vi "SAM.vi"() -> ()   [LabVIEW 2020]
uses:
  <vilib>/Utility/error.llb/DialogType.ctl
  <vilib>/DAQmx/read.llb/DAQmx Read (Analog 1D Wfm NChan NSamp).vi
  <vilib>/DAQmx/create/channels.llb/DAQmx Create Channel (AI-Voltage-Basic).vi
  <vilib>/DAQmx/configure/timing.llb/DAQmx Timing (Sample Clock).vi
  <vilib>/DAQmx/miscellaneous.llb/DAQmx Fill In Error Info.vi
  <vilib>/measure/matone.llb/Harmonic Distortion Analyzer 1 Chan.vi
  <vilib>/express/express analysis/Spectral/Block/exnSpectralBlock spectral measurements RMS poly.vi
  <vilib>/express/express analysis/Spectral/Block/exnSpectralBlock spectral measurements RMS WFM.vi
  <vilib>/measure/madcrms.llb/Basic Averaged DC-RMS for 1 Chan.vi
  <vilib>/measure/matone.llb/Extract Single Tone Information 1 Chan.vi
  <vilib>/express/express analysis/Spectral/XNode/ExpressSpectralMeasurementsBlockNode.xnode
  <resource>/objmgr/daqmx.rc
  <vilib>/measure/NI_MAPro.lvlib
panel:
  out "Voltage":waveform(dbl)(graph)
  out "Uc(Active Power)":dbl
  out "Active Power [W]":dbl
  out "Power":waveform(dbl)(graph)
  out "Phase dif.(V-I)":dbl
  out "THD(V) [dB]":dbl
  out "THD(I) [dB]":dbl
  out "Ih11 [dBA]":dbl
  out "Ih10 [dBA]":dbl
  out "Ih9 [dBA]":dbl
  out "Ih8 [dBA]":dbl
  out "Ih7 [dBA]":dbl
  out "Ih6 [dBA]":dbl
  out "Ih5 [dBA]":dbl
  out "Ih4 [dBA]":dbl
  out "Ih3 [dBA]":dbl
  out "Ih2 [dBA]":dbl
  out "Ih1 [dBA]":dbl
  out "Ih11 [A]":dbl
  out "Ih10 [A]":dbl
  out "Ih9 [A]":dbl
  out "Ih8 [A]":dbl
  out "Ih7 [A]":dbl
  out "Ih6 [A]":dbl
  out "Ih5 [A]":dbl
  out "Ih4 [A]":dbl
  out "Ih3 [A]":dbl
  out "Ih2 [A]":dbl
  out "Ih1 [A]":dbl
  out "fh(I)11 [Hz]":dbl
  out "fh(I)10 [Hz]":dbl
  out "fh(I)9 [Hz]":dbl
  out "fh(I)8 [Hz]":dbl
  out "fh(I)7 [Hz]":dbl
  out "fh(I)6 [Hz]":dbl
  out "fh(I)5 [Hz]":dbl
  out "fh(I)4 [Hz]":dbl
  out "fh(I)3 [Hz]":dbl
  out "fh(I)2 [Hz]":dbl
  out "fh(I)1 [Hz]":dbl
  out "Vh11 [dBV]":dbl
  out "Vh10 [dBV]":dbl
  out "Vh9 [dBV]":dbl
  out "Vh8 [dBV]":dbl
  out "Vh7 [dBV]":dbl
  out "Vh6 [dBV]":dbl
  out "Vh5 [dBV]":dbl
  out "Vh4 [dBV]":dbl
  out "Vh3 [dBV]":dbl
  out "Vh2 [dBV]":dbl
  out "Vh1 [dBV]":dbl
  out "Vh11 [V]":dbl
  out "Vh10 [V]":dbl
  out "Vh9 [V]":dbl
  out "Vh8 [V]":dbl
  out "Vh7 [V]":dbl
  out "Vh6 [V]":dbl
  out "Vh5 [V]":dbl
  out "Vh4 [V]":dbl
  out "Vh3 [V]":dbl
  out "Vh2 [V]":dbl
  out "Vh1 [V]":dbl
  out "fh(V)11 [Hz]":dbl
  out "fh(V)10 [Hz]":dbl
  out "fh(V)9 [Hz]":dbl
  out "fh(V)8 [Hz]":dbl
  out "fh(V)7 [Hz]":dbl
  out "fh(V)6 [Hz]":dbl
  out "fh(V)5 [Hz]":dbl
  out "fh(V)4 [Hz]":dbl
  out "fh(V)3 [Hz]":dbl
  out "fh(V)2 [Hz]":dbl
  out "fh(V)1 [Hz]":dbl
  out "One-sided Spectrum [dbV]":cluster{"f0":dbl, "df":dbl, "magnitude":dbl[]}(graph)
  out "One-sided Spectrum [dbA]":cluster{"f0":dbl, "df":dbl, "magnitude":dbl[]}(graph)
  out "Vrms(I) [A]":dbl
  out "Vm(I) [A]":dbl
  out "Vm(U) [V]":dbl
  out "Vrms(U) [V]":dbl
  out "f(I) [Hz]":dbl
  out "f(U) [Hz]":dbl
  out "Current":waveform(dbl)(graph)
  in  "stop":bool
  in  "Start":bool
  out "Actual sample clk  rate":dbl
  in  "sample clock source":tag
  in  "sample rate":dbl=1000.0 format="%0.2f"
  in  "n of samples":i32=1000
  in  "physical channel":tag
  in  "input terminal configuration":i32(ring)=-1 items=["Default"=-1, "RSE"=10083, "NRSE"=10078, "Differential"=10106, "Pseudodifferential"=12529]
  in  "Min V":dbl=-5.0 format="%0.2f"
  in  "Max V":dbl=5.0 format="%0.2f"
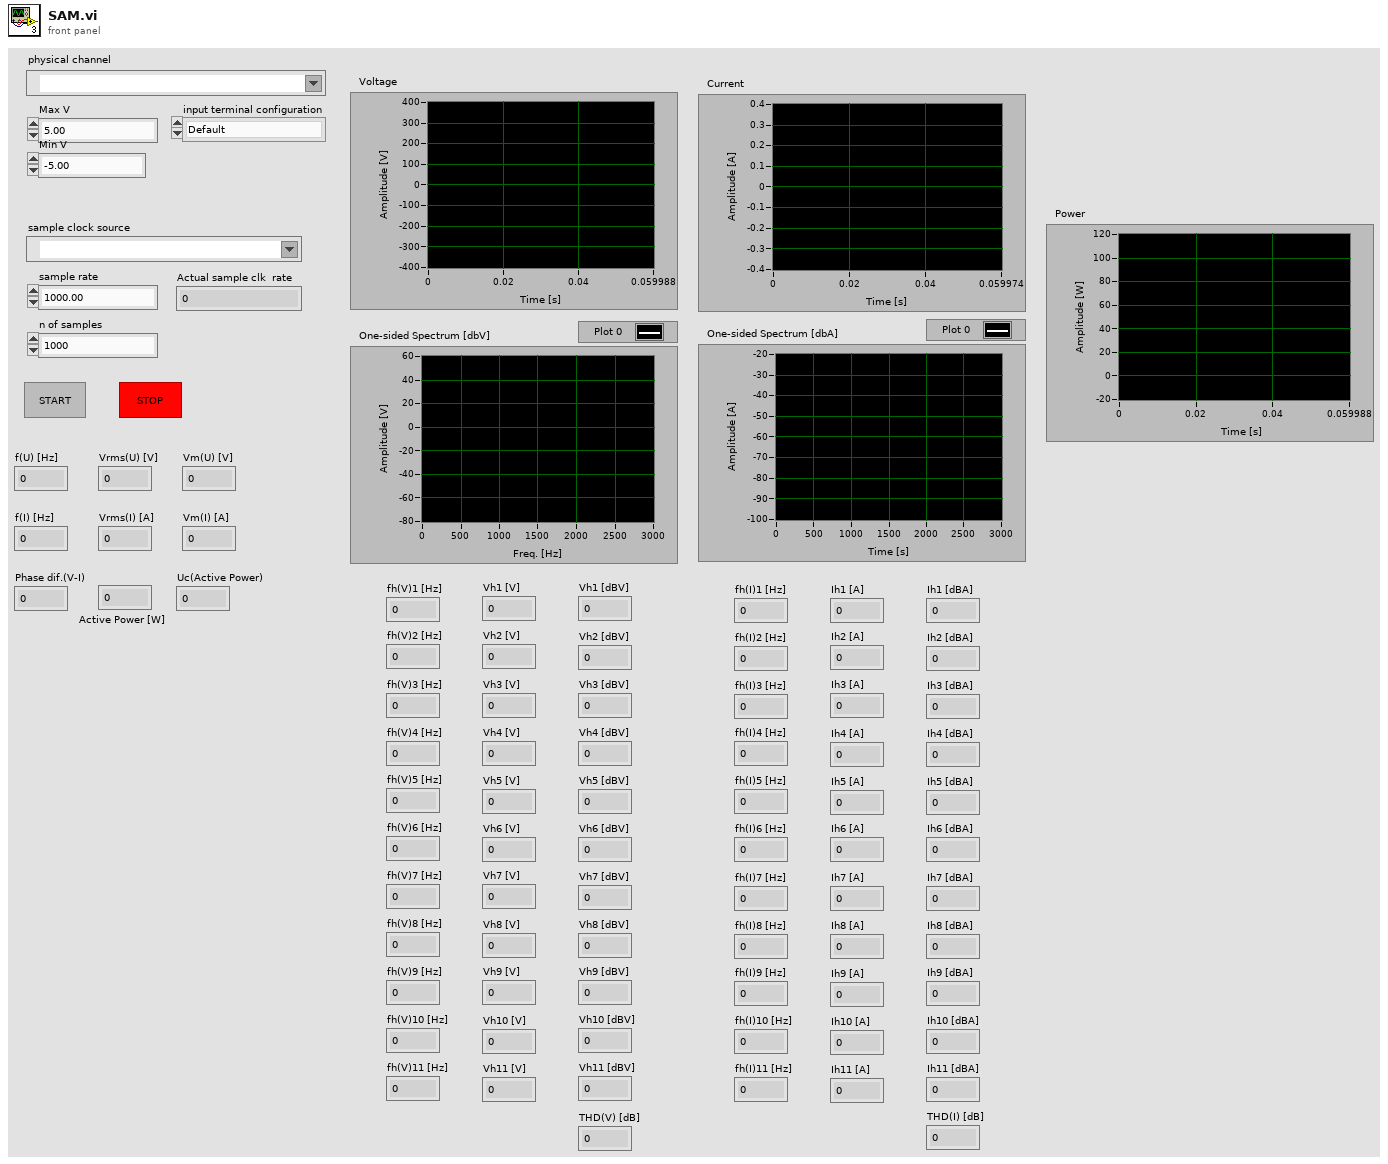
[diagram p1: front panel]
types:
  T1 = typedef "DialogType.ctl" = u16
  T2 = cluster{"averaging mode":u16, "weighting mode":u16, "number of averages":u32}
  T3 = cluster{"dB On (F)":bool, "unwrap phase (F)":bool, "convert to degree (F)":bool}
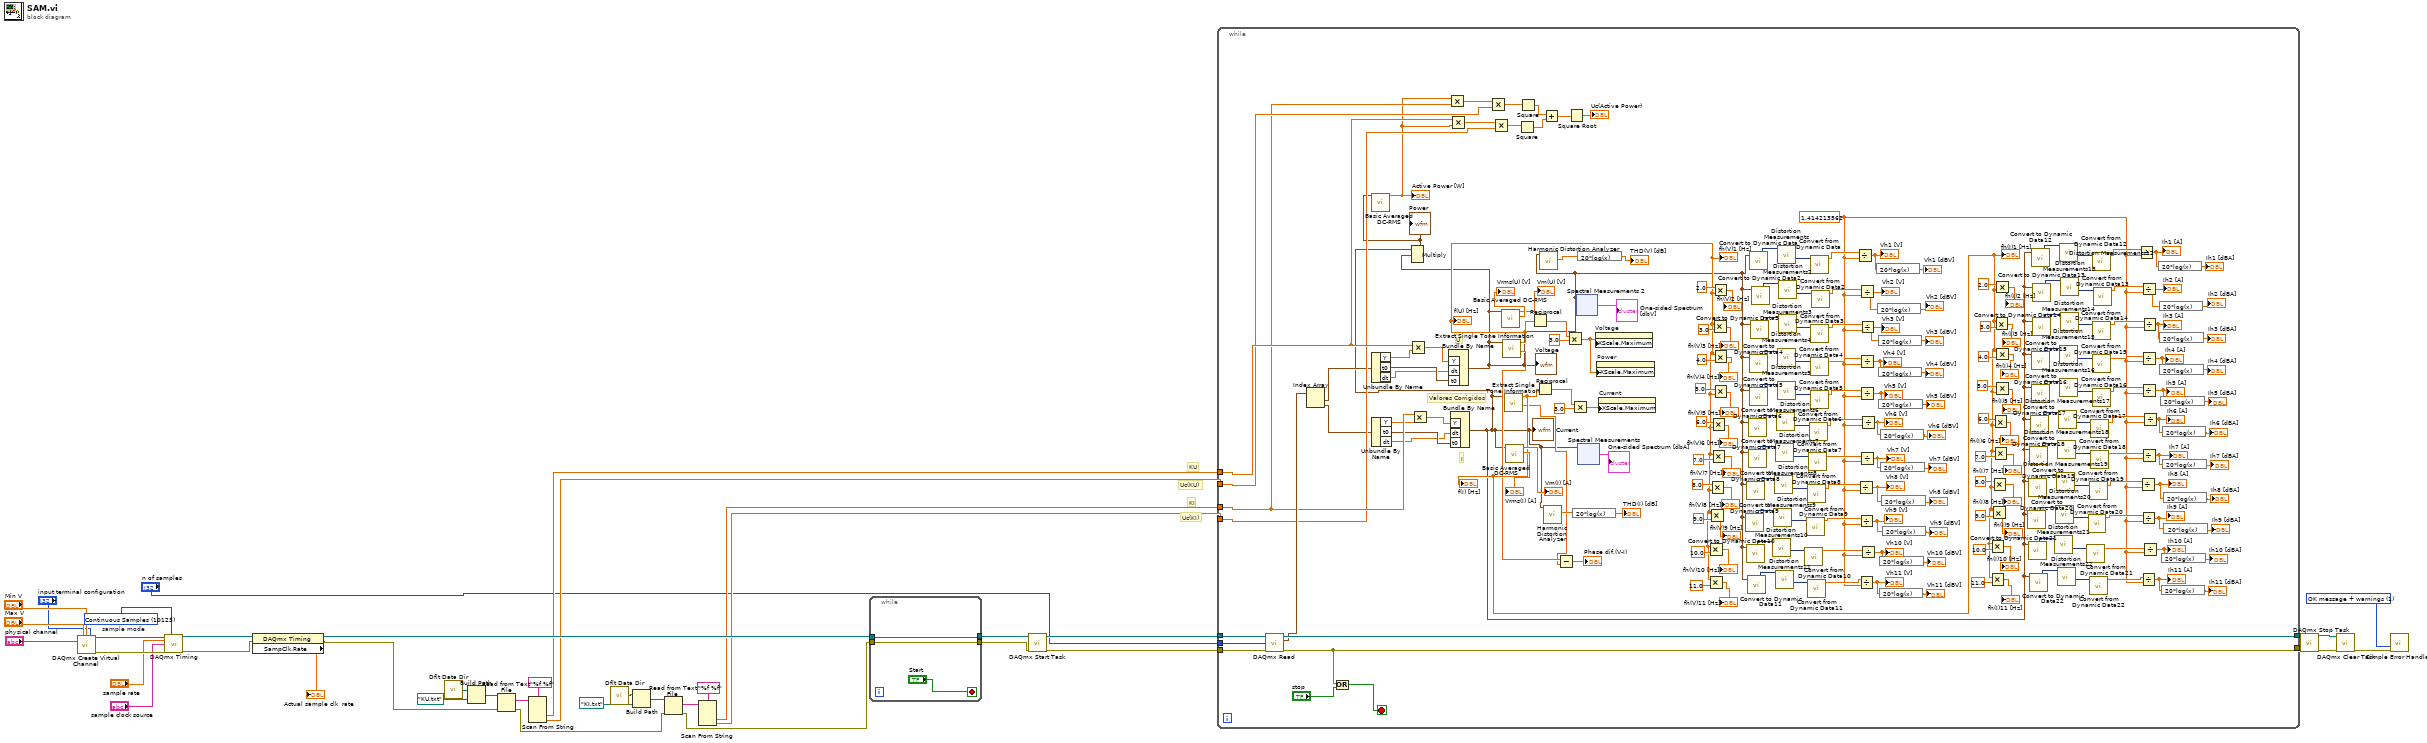
[diagram p0: block diagram]
diagram:
  w27 = T1 1 items=["no dialog", "OK message + warnings", "OK message", "continue or stop message", "continue/stop + warnings"] ("type of dialog (OK msg:1)")
  w33 = 10123 items=["Finite Samples"=10178, "Continuous Samples"=10123, "Hardware Timed Single Point"=12522]  # sample mode
  # "Uc(KU)"
  # "Uc(KI)"
  # "KI"
  # "KU"
  n1 = call-poly <vilib>:"DAQmx Create Virtual Channel.vi"("maximum value"="Max V", "minimum value"="Min V", "input terminal configuration"="input terminal configuration", "physical channels"="physical channel") -> ("task out"=w41:refnum<k21>, "error out"=w40:errorcluster)  [unwired: 10 in]
  n2 = call-poly <vilib>:"DAQmx Timing.vi"("task/channels in"=w41, "sample mode"=w33, "rate"="sample rate", "source"="sample clock source", "error in"=w40) -> ("task out"=w38:refnum<k21>, "error out"=w39:errorcluster)  [unwired: 9 in]
  n3 = property class="DAQmx Timing"(reference=w38, error in=w39) -> (reference out=w25:refnum<k21>, error out=w10:errorcluster, "SampClk.Rate"=→"Actual sample clk  rate":dbl)
  n4 = call <vilib>:"Dflt Data Dir.vi"() -> ("App:Default Data Directory"=w20:path)
  n5 = Build Path(base path=w20, name or relative path=path "KU.txt") -> (appended path=w16:path)
  n6 = Read from Text File(file (use dialog)=w16, error in=w10) -> (text=w17:string, error out=w9:errorcluster)  [unwired: 2 in, 2 out]
  n7 = Scan From String(format string="%f %f", input string=w17) -> (output 1=w7:dbl, output 2=w6:dbl)  [unwired: 4 in, 3 out]
  n8 = call <vilib>:"Dflt Data Dir.vi"() -> ("App:Default Data Directory"=w15:path)
  n9 = Build Path(base path=w15, name or relative path=path "KI.txt") -> (appended path=w11:path)
  n10 = Read from Text File(file (use dialog)=w11, error in=w9) -> (text=w12:string, error out=w8:errorcluster)  [unwired: 2 in, 2 out]
  n11 = Scan From String(format string="%f %f", input string=w12) -> (output 1=w5:dbl, output 2=w4:dbl)  [unwired: 4 in, 3 out]
  n12 = while {
    tunnel: w25 -> [w44]
    tunnel: [w44] -> w24
    tunnel: w8 -> [w43]
    tunnel: [w43] -> w23
    stop <- "Start" stop-if-true
  }
  n13 = call <vilib>:"DAQmx Start Task.vi"("task/channels in"=w24, "error in"=w23) -> ("task out"=w3:refnum<k21>, "error out"=w2:errorcluster)  [unwired: 12 in]
  n14 = while {
    tunnel: [w245] -> w22
    tunnel: [w246] -> w21
    tunnel: w7 -> [w243]
    tunnel: w6 -> [w242]
    tunnel: w5 -> [w241]
    tunnel: w4 -> [w240]
    tunnel: w3 -> [w248]
    tunnel: w2 -> [w247]
    tunnel: "n of samples" -> [w239]
    stop <- w249 stop-if-true
    w69 = 1.414213562 ("x")
    # "I"
    # "U"
    # "Valores Corrigidos"
    n15 = call-poly <vilib>:"DAQmx Read.vi"("task/channels in"=w248, "number of samples per channel"=w239, "error in"=w247) -> ("task out"=w246:refnum<k21>, "data"=w244:waveform(dbl)[], "error out"=w245:errorcluster)  [unwired: 10 in]
    n16 = Index Array(array=w244) -> (element #1=w238:waveform(dbl), element #2=w236:waveform(dbl))  [unwired: 2 in]
    n17 = Or(x=w245, y="stop") -> (x .or. y?=w249:bool)
    n18 = Unbundle By Name(w238) -> ("Y"=w232:dbl[], "t0"=w237:timestamp, "dt"=w233:dbl)
    n19 = Unbundle By Name(w236) -> ("Y"=w231:dbl[], "t0"=w235:timestamp, "dt"=w234:dbl)
    n20 = Multiply(x=w243, y=w232) -> (x*y=w229:dbl[])
    n21 = Multiply(x=w241, y=w231) -> (x*y=w230:dbl[])
    n22 = Bundle By Name("Y"=w229, "dt"=w233, "t0"=w237) -> (w46:waveform(dbl))  [unwired: 1 in]
    "Voltage" <- w46
    n23 = Bundle By Name("Y"=w230, "dt"=w234, "t0"=w235) -> (w59:waveform(dbl))  [unwired: 1 in]
    "Current" <- w59
    n24 = Multiply(1:w46, 2:w59) -> (0:w56:waveform(dbl))  [unwired: 1 in, 1 out]
    "Power" <- w56
    n25 = call-poly <vilib>:"Basic Averaged DC-RMS.vi"("signal in"=w56) -> ("DC value"=w47:dbl)  [unwired: 7 in, 3 out]
    "Active Power [W]" <- w47
    n26 = Multiply(x=w47, y=w241) -> (x*y=w49:dbl)
    n27 = Multiply(x=w243, y=w47) -> (x*y=w48:dbl)
    n28 = Multiply(x=w49, y=w242) -> (x*y=w51:dbl)
    n29 = Multiply(x=w48, y=w240) -> (x*y=w50:dbl)
    n30 = call-poly <vilib>:"Basic Averaged DC-RMS.vi"("signal in"=w46) -> ("RMS value"=→"Vrms(U) [V]":dbl, "DC value"=→"Vm(U) [V]":dbl)  [unwired: 7 in, 2 out]
    n31 = call-poly <vilib>:"Extract Single Tone Information.vi"("time signal in"=w46) -> ("detected phase (deg)"=w62:dbl, "detected frequency"=w185:dbl)  [unwired: 5 in, 4 out]
    "f(U) [Hz]" <- w185
    "fh(V)1 [Hz]" <- w185
    n32 = call-poly <vilib>:"Extract Single Tone Information.vi"("time signal in"=w59) -> ("detected phase (deg)"=w61:dbl, "detected frequency"=w68:dbl)  [unwired: 5 in, 4 out]
    "f(I) [Hz]" <- w68
    "fh(I)1 [Hz]" <- w68
    n33 = call-poly <vilib>:"Basic Averaged DC-RMS.vi"("signal in"=w59) -> ("RMS value"=→"Vrms(I) [A]":dbl, "DC value"=→"Vm(I) [A]":dbl)  [unwired: 7 in, 2 out]
    n34 = Square(x=w50) -> (x^2=w52:dbl)
    n35 = Square(x=w51) -> (x^2=w53:dbl)
    n36 = Reciprocal(x=w185) -> (1/x=w228:dbl)
    n37 = Reciprocal(x=w68) -> (1/x=w226:dbl)
    n38 = call-poly <vilib>:"Harmonic Distortion Analyzer.vi"("signal in"=w46) -> ("THD"=w67:dbl)  [unwired: 5 in, 5 out]
    n39 = Add(x=w53, y=w52) -> (x+y=w54:dbl)
    n40 = call-poly <vilib>:"Harmonic Distortion Analyzer.vi"("signal in"=w59) -> ("THD"=w66:dbl)  [unwired: 5 in, 5 out]
    n41 = Subtract(x=w62, y=w61) -> (x-y=→"Phase dif.(V-I)":dbl)
    n42 = Multiply(x=w228, y=3.0 ("x*y")) -> (x*y=w45:dbl)
    n43 = Square Root(x=w54) -> (sqrt(x)=→"Uc(Active Power)":dbl)
    n44 = Multiply(x=w226, y=3.0 ("x*y")) -> (x*y=w224:dbl)
    n45 = expression code="20*log(x)"(w66) -> (→"THD(I) [dB]":dbl)
    n46 = xnode "Spectral Measurements 2"("Signals"=w46) -> ("FFT - (RMS)"=→"One-sided Spectrum [dbV]":cluster{"f0":dbl, "df":dbl, "magnitude":dbl[]})  [unwired: 1 in, 2 out]
    n47 = expression code="20*log(x)"(w67) -> (→"THD(V) [dB]":dbl)
    n48 = xnode "Spectral Measurements"("Signals"=w59) -> ("FFT - (RMS)"=→"One-sided Spectrum [dbA]":cluster{"f0":dbl, "df":dbl, "magnitude":dbl[]})  [unwired: 1 in, 2 out]
    n49 = property on="Voltage" class="WFGraph (strict)"("XScale.Maximum"=w45) -> ()  [unwired: 2 in, 2 out]
    n50 = property on="Power" class="WFGraph (strict)"("XScale.Maximum"=w45) -> ()  [unwired: 2 in, 2 out]
    n51 = property on="Current" class="WFGraph (strict)"("XScale.Maximum"=w224) -> ()  [unwired: 2 in, 2 out]
    n52 = Multiply(x=w185, y=10.0) -> (x*y=→"fh(V)10 [Hz]":dbl)
    n53 = Multiply(x=w185, y=11.0) -> (x*y=→"fh(V)11 [Hz]":dbl)
    n54 = Multiply(x=w185, y=9.0 ("x*y")) -> (x*y=→"fh(V)9 [Hz]":dbl)
    n55 = Multiply(x=8.0, y=w185) -> (x*y=→"fh(V)8 [Hz]":dbl)
    n56 = Multiply(x=6.0 ("x*y"), y=w185) -> (x*y=→"fh(V)6 [Hz]":dbl)
    n57 = Multiply(x=w185, y=7.0) -> (x*y=→"fh(V)7 [Hz]":dbl)
    n58 = Multiply(x=w185, y=3.0 ("x*y")) -> (x*y=→"fh(V)3 [Hz]":dbl)
    n59 = Multiply(x=2.0, y=w185) -> (x*y=→"fh(V)2 [Hz]":dbl)
    n60 = Multiply(x=w185, y=4.0 ("x*y")) -> (x*y=→"fh(V)4 [Hz]":dbl)
    n61 = Multiply(x=5.0, y=w185) -> (x*y=→"fh(V)5 [Hz]":dbl)
    n62 = call "Convert to Dynamic Data9"("Waveform"=w46) -> ("Dynamic Data Type"=w201:dynamicdata)  [unwired: 3 in]
    n63 = call "Convert to Dynamic Data10"("Waveform"=w46) -> ("Dynamic Data Type"=w198:dynamicdata)  [unwired: 3 in]
    n64 = call "Convert to Dynamic Data8"("Waveform"=w46) -> ("Dynamic Data Type"=w202:dynamicdata)  [unwired: 3 in]
    n65 = call "Convert to Dynamic Data11"("Waveform"=w46) -> ("Dynamic Data Type"=w197:dynamicdata)  [unwired: 3 in]
    n66 = call "Convert to Dynamic Data7"("Waveform"=w46) -> ("Dynamic Data Type"=w205:dynamicdata)  [unwired: 3 in]
    n67 = call "Convert to Dynamic Data6"("Waveform"=w46) -> ("Dynamic Data Type"=w206:dynamicdata)  [unwired: 3 in]
    n68 = call "Convert to Dynamic Data"("Waveform"=w46) -> ("Dynamic Data Type"=w217:dynamicdata)  [unwired: 3 in]
    n69 = call "Convert to Dynamic Data4"("Waveform"=w46) -> ("Dynamic Data Type"=w210:dynamicdata)  [unwired: 3 in]
    n70 = call "Convert to Dynamic Data5"("Waveform"=w46) -> ("Dynamic Data Type"=w209:dynamicdata)  [unwired: 3 in]
    n71 = call "Convert to Dynamic Data3"("Waveform"=w46) -> ("Dynamic Data Type"=w213:dynamicdata)  [unwired: 3 in]
    n72 = call "Convert to Dynamic Data2"("Waveform"=w46) -> ("Dynamic Data Type"=w214:dynamicdata)  [unwired: 3 in]
    n73 = call "Distortion Measurements10"("Signals"=w198) -> ("Specific Harmonic"=w199:dynamicdata)  [unwired: 9 in, 1 out]
    n74 = call "Distortion Measurements9"("Signals"=w201) -> ("Specific Harmonic"=w200:dynamicdata)  [unwired: 9 in, 1 out]
    n75 = call "Distortion Measurements8"("Signals"=w202) -> ("Specific Harmonic"=w203:dynamicdata)  [unwired: 9 in, 1 out]
    n76 = call "Distortion Measurements11"("Signals"=w197) -> ("Specific Harmonic"=w196:dynamicdata)  [unwired: 9 in, 1 out]
    n77 = call "Distortion Measurements7"("Signals"=w205) -> ("Specific Harmonic"=w204:dynamicdata)  [unwired: 9 in, 1 out]
    n78 = call "Distortion Measurements6"("Signals"=w206) -> ("Specific Harmonic"=w207:dynamicdata)  [unwired: 9 in, 1 out]
    n79 = call "Distortion Measurements"("Signals"=w217) -> ("Specific Harmonic"=w216:dynamicdata)  [unwired: 9 in, 1 out]
    n80 = call "Distortion Measurements4"("Signals"=w210) -> ("Specific Harmonic"=w211:dynamicdata)  [unwired: 9 in, 1 out]
    n81 = call "Distortion Measurements5"("Signals"=w209) -> ("Specific Harmonic"=w208:dynamicdata)  [unwired: 9 in, 1 out]
    n82 = call "Distortion Measurements3"("Signals"=w213) -> ("Specific Harmonic"=w212:dynamicdata)  [unwired: 9 in, 1 out]
    n83 = call "Distortion Measurements2"("Signals"=w214) -> ("Specific Harmonic"=w215:dynamicdata)  [unwired: 9 in, 1 out]
    n84 = call "Convert from Dynamic Data10"("Dynamic Data Type"=w199) -> ("Scalar"=w165:dbl)  [unwired: 3 in]
    n85 = call "Convert from Dynamic Data9"("Dynamic Data Type"=w200) -> ("Scalar"=w166:dbl)  [unwired: 3 in]
    n86 = call "Convert from Dynamic Data8"("Dynamic Data Type"=w203) -> ("Scalar"=w167:dbl)  [unwired: 3 in]
    n87 = call "Convert from Dynamic Data11"("Dynamic Data Type"=w196) -> ("Scalar"=w164:dbl)  [unwired: 3 in]
    n88 = call "Convert from Dynamic Data7"("Dynamic Data Type"=w204) -> ("Scalar"=w168:dbl)  [unwired: 3 in]
    n89 = call "Convert from Dynamic Data6"("Dynamic Data Type"=w207) -> ("Scalar"=w169:dbl)  [unwired: 3 in]
    n90 = call "Convert from Dynamic Data"("Dynamic Data Type"=w216) -> ("Scalar"=w174:dbl)  [unwired: 3 in]
    n91 = call "Convert from Dynamic Data4"("Dynamic Data Type"=w211) -> ("Scalar"=w171:dbl)  [unwired: 3 in]
    n92 = call "Convert from Dynamic Data5"("Dynamic Data Type"=w208) -> ("Scalar"=w170:dbl)  [unwired: 3 in]
    n93 = call "Convert from Dynamic Data3"("Dynamic Data Type"=w212) -> ("Scalar"=w172:dbl)  [unwired: 3 in]
    n94 = call "Convert from Dynamic Data2"("Dynamic Data Type"=w215) -> ("Scalar"=w173:dbl)  [unwired: 3 in]
    n95 = Divide(x=w174, y=w69) -> (x/y=w163:dbl)
    "Vh1 [V]" <- w163
    n96 = Divide(x=w167, y=w69) -> (x/y=w57:dbl)
    "Vh8 [V]" <- w57
    n97 = Divide(x=w166, y=w69) -> (x/y=w152:dbl)
    "Vh9 [V]" <- w152
    n98 = Divide(x=w164, y=w69) -> (x/y=w150:dbl)
    "Vh11 [V]" <- w150
    n99 = Divide(x=w173, y=w69) -> (x/y=w160:dbl)
    "Vh2 [V]" <- w160
    n100 = Divide(x=w171, y=w69) -> (x/y=w156:dbl)
    "Vh4 [V]" <- w156
    n101 = Divide(x=w170, y=w69) -> (x/y=w154:dbl)
    "Vh5 [V]" <- w154
    n102 = Divide(x=w168, y=w69) -> (x/y=w153:dbl)
    "Vh7 [V]" <- w153
    n103 = Divide(x=w172, y=w69) -> (x/y=w158:dbl)
    "Vh3 [V]" <- w158
    n104 = Divide(x=w169, y=w69) -> (x/y=w149:dbl)
    "Vh6 [V]" <- w149
    n105 = Divide(x=w165, y=w69) -> (x/y=w151:dbl)
    "Vh10 [V]" <- w151
    n106 = expression code="20*log(x)"(w163) -> (→"Vh1 [dBV]":dbl)
    n107 = expression code="20*log(x)"(w160) -> (→"Vh2 [dBV]":dbl)
    n108 = expression code="20*log(x)"(w158) -> (→"Vh3 [dBV]":dbl)
    n109 = expression code="20*log(x)"(w156) -> (→"Vh4 [dBV]":dbl)
    n110 = expression code="20*log(x)"(w154) -> (→"Vh5 [dBV]":dbl)
    n111 = expression code="20*log(x)"(w150) -> (→"Vh11 [dBV]":dbl)
    n112 = expression code="20*log(x)"(w151) -> (→"Vh10 [dBV]":dbl)
    n113 = expression code="20*log(x)"(w149) -> (→"Vh6 [dBV]":dbl)
    n114 = expression code="20*log(x)"(w153) -> (→"Vh7 [dBV]":dbl)
    n115 = expression code="20*log(x)"(w57) -> (→"Vh8 [dBV]":dbl)
    n116 = expression code="20*log(x)"(w152) -> (→"Vh9 [dBV]":dbl)
    n117 = Multiply(x=w68, y=10.0) -> (x*y=→"fh(I)10 [Hz]":dbl)
    n118 = Multiply(x=w68, y=11.0) -> (x*y=→"fh(I)11 [Hz]":dbl)
    n119 = Multiply(x=w68, y=9.0 ("x*y")) -> (x*y=→"fh(I)9 [Hz]":dbl)
    n120 = Multiply(x=8.0 ("y"), y=w68) -> (x*y=→"fh(I)8 [Hz]":dbl)
    n121 = Multiply(x=6.0 ("x*y"), y=w68) -> (x*y=→"fh(I)6 [Hz]":dbl)
    n122 = Multiply(x=w68, y=7.0) -> (x*y=→"fh(I)7 [Hz]":dbl)
    n123 = Multiply(x=w68, y=3.0 ("x*y")) -> (x*y=→"fh(I)3 [Hz]":dbl)
    n124 = Multiply(x=2.0, y=w68) -> (x*y=→"fh(I)2 [Hz]":dbl)
    n125 = Multiply(x=w68, y=4.0 ("x*y")) -> (x*y=→"fh(I)4 [Hz]":dbl)
    n126 = Multiply(x=5.0, y=w68) -> (x*y=→"fh(I)5 [Hz]":dbl)
    n127 = call "Convert to Dynamic Data20"("Waveform"=w59) -> ("Dynamic Data Type"=w126:dynamicdata)  [unwired: 3 in]
    n128 = call "Convert to Dynamic Data21"("Waveform"=w59) -> ("Dynamic Data Type"=w123:dynamicdata)  [unwired: 3 in]
    n129 = call "Convert to Dynamic Data19"("Waveform"=w59) -> ("Dynamic Data Type"=w127:dynamicdata)  [unwired: 3 in]
    n130 = call "Convert to Dynamic Data22"("Waveform"=w59) -> ("Dynamic Data Type"=w122:dynamicdata)  [unwired: 3 in]
    n131 = call "Convert to Dynamic Data18"("Waveform"=w59) -> ("Dynamic Data Type"=w130:dynamicdata)  [unwired: 3 in]
    n132 = call "Convert to Dynamic Data17"("Waveform"=w59) -> ("Dynamic Data Type"=w131:dynamicdata)  [unwired: 3 in]
    n133 = call "Convert to Dynamic Data12"("Waveform"=w59) -> ("Dynamic Data Type"=w142:dynamicdata)  [unwired: 3 in]
    n134 = call "Convert to Dynamic Data15"("Waveform"=w59) -> ("Dynamic Data Type"=w135:dynamicdata)  [unwired: 3 in]
    n135 = call "Convert to Dynamic Data16"("Waveform"=w59) -> ("Dynamic Data Type"=w134:dynamicdata)  [unwired: 3 in]
    n136 = call "Convert to Dynamic Data14"("Waveform"=w59) -> ("Dynamic Data Type"=w138:dynamicdata)  [unwired: 3 in]
    n137 = call "Convert to Dynamic Data13"("Waveform"=w59) -> ("Dynamic Data Type"=w139:dynamicdata)  [unwired: 3 in]
    n138 = call "Distortion Measurements21"("Signals"=w123) -> ("Specific Harmonic"=w124:dynamicdata)  [unwired: 9 in, 1 out]
    n139 = call "Distortion Measurements20"("Signals"=w126) -> ("Specific Harmonic"=w125:dynamicdata)  [unwired: 9 in, 1 out]
    n140 = call "Distortion Measurements19"("Signals"=w127) -> ("Specific Harmonic"=w128:dynamicdata)  [unwired: 9 in, 1 out]
    n141 = call "Distortion Measurements22"("Signals"=w122) -> ("Specific Harmonic"=w121:dynamicdata)  [unwired: 9 in, 1 out]
    n142 = call "Distortion Measurements18"("Signals"=w130) -> ("Specific Harmonic"=w129:dynamicdata)  [unwired: 9 in, 1 out]
    n143 = call "Distortion Measurements17"("Signals"=w131) -> ("Specific Harmonic"=w132:dynamicdata)  [unwired: 9 in, 1 out]
    n144 = call "Distortion Measurements12"("Signals"=w142) -> ("Specific Harmonic"=w141:dynamicdata)  [unwired: 9 in, 1 out]
    n145 = call "Distortion Measurements15"("Signals"=w135) -> ("Specific Harmonic"=w136:dynamicdata)  [unwired: 9 in, 1 out]
    n146 = call "Distortion Measurements16"("Signals"=w134) -> ("Specific Harmonic"=w133:dynamicdata)  [unwired: 9 in, 1 out]
    n147 = call "Distortion Measurements14"("Signals"=w138) -> ("Specific Harmonic"=w137:dynamicdata)  [unwired: 9 in, 1 out]
    n148 = call "Distortion Measurements13"("Signals"=w139) -> ("Specific Harmonic"=w140:dynamicdata)  [unwired: 9 in, 1 out]
    n149 = call "Convert from Dynamic Data21"("Dynamic Data Type"=w124) -> ("Scalar"=w92:dbl)  [unwired: 3 in]
    n150 = call "Convert from Dynamic Data20"("Dynamic Data Type"=w125) -> ("Scalar"=w93:dbl)  [unwired: 3 in]
    n151 = call "Convert from Dynamic Data19"("Dynamic Data Type"=w128) -> ("Scalar"=w94:dbl)  [unwired: 3 in]
    n152 = call "Convert from Dynamic Data22"("Dynamic Data Type"=w121) -> ("Scalar"=w91:dbl)  [unwired: 3 in]
    n153 = call "Convert from Dynamic Data18"("Dynamic Data Type"=w129) -> ("Scalar"=w95:dbl)  [unwired: 3 in]
    n154 = call "Convert from Dynamic Data17"("Dynamic Data Type"=w132) -> ("Scalar"=w96:dbl)  [unwired: 3 in]
    n155 = call "Convert from Dynamic Data12"("Dynamic Data Type"=w141) -> ("Scalar"=w101:dbl)  [unwired: 3 in]
    n156 = call "Convert from Dynamic Data15"("Dynamic Data Type"=w136) -> ("Scalar"=w98:dbl)  [unwired: 3 in]
    n157 = call "Convert from Dynamic Data16"("Dynamic Data Type"=w133) -> ("Scalar"=w97:dbl)  [unwired: 3 in]
    n158 = call "Convert from Dynamic Data14"("Dynamic Data Type"=w137) -> ("Scalar"=w99:dbl)  [unwired: 3 in]
    n159 = call "Convert from Dynamic Data13"("Dynamic Data Type"=w140) -> ("Scalar"=w100:dbl)  [unwired: 3 in]
    n160 = Divide(x=w101, y=w69) -> (x/y=w90:dbl)
    "Ih1 [A]" <- w90
    n161 = Divide(x=w94, y=w69) -> (x/y=w58:dbl)
    "Ih8 [A]" <- w58
    n162 = Divide(x=w93, y=w69) -> (x/y=w79:dbl)
    "Ih9 [A]" <- w79
    n163 = Divide(x=w91, y=w69) -> (x/y=w77:dbl)
    "Ih11 [A]" <- w77
    n164 = Divide(x=w100, y=w69) -> (x/y=w87:dbl)
    "Ih2 [A]" <- w87
    n165 = Divide(x=w98, y=w69) -> (x/y=w83:dbl)
    "Ih4 [A]" <- w83
    n166 = Divide(x=w97, y=w69) -> (x/y=w81:dbl)
    "Ih5 [A]" <- w81
    n167 = Divide(x=w95, y=w69) -> (x/y=w80:dbl)
    "Ih7 [A]" <- w80
    n168 = Divide(x=w99, y=w69) -> (x/y=w85:dbl)
    "Ih3 [A]" <- w85
    n169 = Divide(x=w96, y=w69) -> (x/y=w76:dbl)
    "Ih6 [A]" <- w76
    n170 = Divide(x=w92, y=w69) -> (x/y=w78:dbl)
    "Ih10 [A]" <- w78
    n171 = expression code="20*log(x)"(w90) -> (→"Ih1 [dBA]":dbl)
    n172 = expression code="20*log(x)"(w87) -> (→"Ih2 [dBA]":dbl)
    n173 = expression code="20*log(x)"(w85) -> (→"Ih3 [dBA]":dbl)
    n174 = expression code="20*log(x)"(w83) -> (→"Ih4 [dBA]":dbl)
    n175 = expression code="20*log(x)"(w81) -> (→"Ih5 [dBA]":dbl)
    n176 = expression code="20*log(x)"(w77) -> (→"Ih11 [dBA]":dbl)
    n177 = expression code="20*log(x)"(w78) -> (→"Ih10 [dBA]":dbl)
    n178 = expression code="20*log(x)"(w76) -> (→"Ih6 [dBA]":dbl)
    n179 = expression code="20*log(x)"(w80) -> (→"Ih7 [dBA]":dbl)
    n180 = expression code="20*log(x)"(w58) -> (→"Ih8 [dBA]":dbl)
    n181 = expression code="20*log(x)"(w79) -> (→"Ih9 [dBA]":dbl)
  }
  n182 = call <vilib>:"DAQmx Stop Task.vi"("task/channels in"=w21, "error in"=w22) -> ("task out"=w30:refnum<k21>, "error out"=w29:errorcluster)  [unwired: 12 in]
  n183 = call <vilib>:"DAQmx Clear Task.vi"("task in"=w30, "error in"=w29) -> ("error out"=w28:errorcluster)  [unwired: 13 in]
  n184 = call <vilib>:"Simple Error Handler.vi"("type of dialog (OK msg:1)"=w27, "error in (no error)"=w28) -> ()  [unwired: 3 in, 5 out]
